vi "Overlay Tips.vi"(6 "Color":u32(colorbox)=6618880, 8 "error in (no error)":errorcluster, 9 "Image Array":T1[](array[typedef]), 10 "Tips":T2[](array[typedef]) {"Point"."Y" format="%.2f"; "Point"."X" format="%.2f"}, 11 "Image":T1) -> (0 "error out":errorcluster, 2 "Tips out":T2[](array[typedef]) {"Point"."Y" format="%.2f"; "Point"."X" format="%.2f"}, 3 "Image Out":T1)   [LabVIEW 2013]
uses:
  Controls/Tip.ctl
  <vilib>/vision/Image Controls.llb/IMAQ Image.ctl
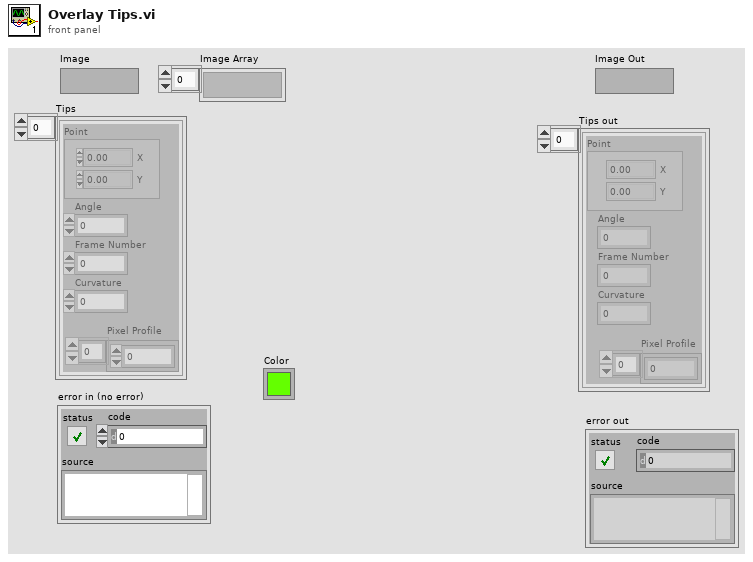
[diagram p1: front panel]
types:
  T1 = typedef "IMAQ Image.ctl" = refnum<image>
  T2 = typedef "Tip.ctl" = cluster{"Point":T3, "Angle":dbl, "Frame Number":i32, "Curvature":dbl, "Pixel Profile":dbl[]}
  T3 = typedef "IMAQ Point" = cluster{"X":sgl, "Y":sgl}
  T4 = cluster{"Left":i32, "Top":i32, "Right":i32, "Bottom":i32}
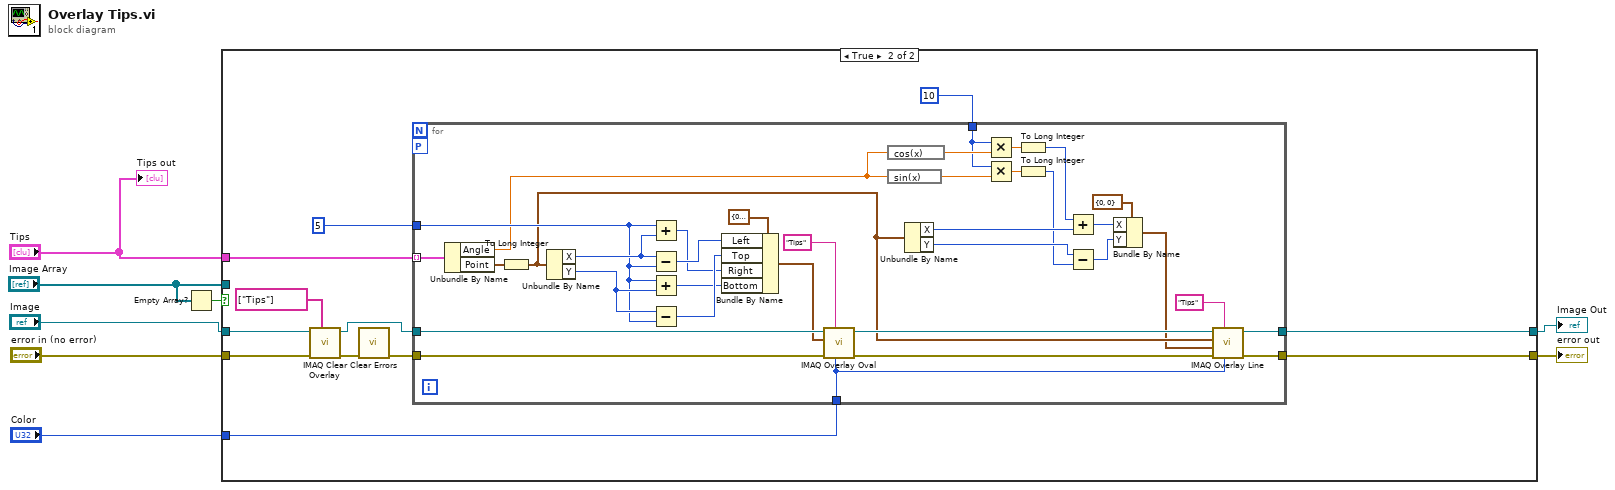
[diagram p0: block diagram]
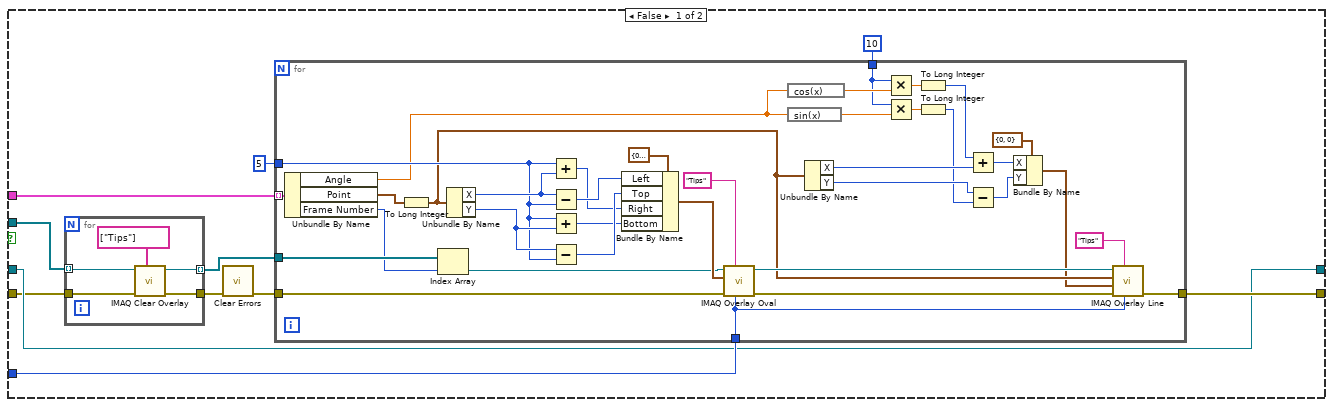
[diagram p2: hidden frame]
diagram:
  n1 = Empty Array?(array="Image Array") -> (empty?=w2:bool)
  n2 = case shown="True" w2 {
    tunnel: [w14 w70] -> w8
    tunnel: [w15 w69] -> w7
    tunnel: "Tips" -> [w18 w68]
    tunnel: "Color" -> [w16 w67]
    tunnel: "error in (no error)" -> [w13 w66]
    tunnel: "Image" -> [w14 w65]
    tunnel: "Image Array" -> [w12 _]
    frame False {
      n3 = for {
        tunnel: w13 -> [w23]
        tunnel: w12 -> [w22] mode=indexing
        tunnel: [w21] -> w11
        tunnel: [w20] -> w9 mode=indexing
        n4 = call "IMAQ Clear Overlay"("Groups"=string[] ["Tips"], "error in (no error)"=w23, "Image"=w22) -> ("error out"=w21:errorcluster, "Image Out"=w20:T1)  [unwired: 7 in]
      }
      n5 = call <vilib>:"Clear Errors.vi"("error in (no error)"=w11) -> ("error out"=w10:errorcluster)  [unwired: 6 in]
      n6 = for {
        tunnel: w10 -> [w50]
        tunnel: w18 -> [w60] mode=indexing
        tunnel: 5 -> [w56]
        tunnel: 10 -> [w43]
        tunnel: [w32] -> w15
        tunnel: w16 -> [w31]
        tunnel: w9 -> [w27]
        n7 = Unbundle By Name(w60) -> ("Angle"=w30:dbl, "Point"=w59:T3, "Frame Number"=w26:i32)
        n8 = To Long Integer(number=w59) -> (32bit integer=w42:cluster{"X":i32, "Y":i32})
        n9 = Index Array(array=w27, index=w26) -> (element=w25:T1)
        n10 = Unbundle By Name(w42) -> ("X"=w58:i32, "Y"=w57:i32)
        n11 = Add(x=w56, y=w58) -> (x+y=w52:i32)
        n12 = Subtract(x=w58, y=w56) -> (x-y=w54:i32)
        n13 = Add(x=w56, y=w57) -> (x+y=w51:i32)
        n14 = Subtract(x=w57, y=w56) -> (x-y=w53:i32)
        n15 = Bundle By Name(cluster=T4 {"Left"=0, "Top"=0, "Right"=0, "Bottom"=0} ("Bounding Rectangle"), "Left"=w54, "Top"=w53, "Right"=w52, "Bottom"=w51) -> (w49:T4)
        n16 = call "IMAQ Overlay Oval"("Color"=w31, "Group"="Tips", "error in (no error)"=w50, "Bounding Rectangle"=w49, "Image"=w25) -> ("error out"=w48:errorcluster, "Image Out"=w47:T1)  [unwired: 5 in]
        n17 = expression code="cos(x)"(w30) -> (w45:dbl)
        n18 = expression code="sin(x)"(w30) -> (w44:dbl)
        n19 = Unbundle By Name(w42) -> ("X"=w41:i32, "Y"=w29:i32)
        n20 = Multiply(x=w43, y=w45) -> (x*y=w40:dbl)
        n21 = Multiply(x=w43, y=w44) -> (x*y=w39:dbl)
        n22 = To Long Integer(number=w40) -> (32bit integer=w38:i32)
        n23 = To Long Integer(number=w39) -> (32bit integer=w28:i32)
        n24 = Add(x=w38, y=w41) -> (x+y=w37:i32)
        n25 = Subtract(x=w29, y=w28) -> (x-y=w36:i32)
        n26 = Bundle By Name(cluster=cluster{"X":i32, "Y":i32} {"X"=0, "Y"=0} ("32bit integer"), "X"=w37, "Y"=w36) -> (w35:cluster{"X":i32, "Y":i32})
        n27 = call "IMAQ Overlay Line"("Color"=w31, "Group"="Tips", "error in (no error)"=w48, "End Point"=w35, "Start Point"=w42, "Image"=w47) -> ("error out"=w32:errorcluster)  [unwired: 4 in, 1 out]
      }
    }
    frame True {
      n28 = call "IMAQ Clear Overlay"("Groups"=string[] ["Tips"], "error in (no error)"=w66, "Image"=w65) -> ("error out"=w63:errorcluster, "Image Out"=w61:T1)  [unwired: 7 in]
      n29 = call <vilib>:"Clear Errors.vi"("error in (no error)"=w63) -> ("error out"=w62:errorcluster)  [unwired: 6 in]
      n30 = for {
        tunnel: w62 -> [w97]
        tunnel: w68 -> [w107] mode=indexing
        tunnel: 5 -> [w103]
        tunnel: w61 -> [w96]
        tunnel: 10 -> [w89]
        tunnel: [w78] -> w70
        tunnel: [w77] -> w69
        tunnel: w67 -> [w76]
        workers-P: _ -> [_]
        n31 = Unbundle By Name(w107) -> ("Angle"=w75:dbl, "Point"=w106:T3)
        n32 = To Long Integer(number=w106) -> (32bit integer=w88:cluster{"X":i32, "Y":i32})
        n33 = Unbundle By Name(w88) -> ("X"=w105:i32, "Y"=w104:i32)
        n34 = Add(x=w103, y=w105) -> (x+y=w99:i32)
        n35 = Subtract(x=w105, y=w103) -> (x-y=w101:i32)
        n36 = Add(x=w103, y=w104) -> (x+y=w98:i32)
        n37 = Subtract(x=w104, y=w103) -> (x-y=w100:i32)
        n38 = Bundle By Name(cluster=T4 {"Left"=0, "Top"=0, "Right"=0, "Bottom"=0} ("Bounding Rectangle"), "Left"=w101, "Top"=w100, "Right"=w99, "Bottom"=w98) -> (w95:T4)
        n39 = call "IMAQ Overlay Oval"("Color"=w76, "Group"="Tips", "error in (no error)"=w97, "Bounding Rectangle"=w95, "Image"=w96) -> ("error out"=w94:errorcluster, "Image Out"=w93:T1)  [unwired: 5 in]
        n40 = expression code="cos(x)"(w75) -> (w91:dbl)
        n41 = expression code="sin(x)"(w75) -> (w90:dbl)
        n42 = Unbundle By Name(w88) -> ("X"=w87:i32, "Y"=w74:i32)
        n43 = Multiply(x=w89, y=w91) -> (x*y=w86:dbl)
        n44 = Multiply(x=w89, y=w90) -> (x*y=w85:dbl)
        n45 = To Long Integer(number=w86) -> (32bit integer=w84:i32)
        n46 = To Long Integer(number=w85) -> (32bit integer=w73:i32)
        n47 = Add(x=w84, y=w87) -> (x+y=w83:i32)
        n48 = Subtract(x=w74, y=w73) -> (x-y=w82:i32)
        n49 = Bundle By Name(cluster=cluster{"X":i32, "Y":i32} {"X"=0, "Y"=0} ("32bit integer"), "X"=w83, "Y"=w82) -> (w81:cluster{"X":i32, "Y":i32})
        n50 = call "IMAQ Overlay Line"("Color"=w76, "Group"="Tips", "error in (no error)"=w94, "End Point"=w81, "Start Point"=w88, "Image"=w93) -> ("error out"=w77:errorcluster, "Image Out"=w78:T1)  [unwired: 4 in]
      }
    }
  }
  "Image Out" <- w8
  "error out" <- w7
  "Tips out" <- "Tips"
